vi "Stop.vi"(8 "error in (no error)":errorcluster, 11 "Virt Instr Target in":refnum<class "Virt Instr Target.lvclass">) -> (0 "error out":errorcluster, 3 "Virt Instr Target out":refnum<class "Virt Instr Target.lvclass">)   [LabVIEW 2023, in "HAL GOOP4.lvlib" / "Virt Instr Target.lvclass"]
uses:
  Virt Instr Target.lvclass
  Virt Instr Host/Virt Instr Host.lvclass
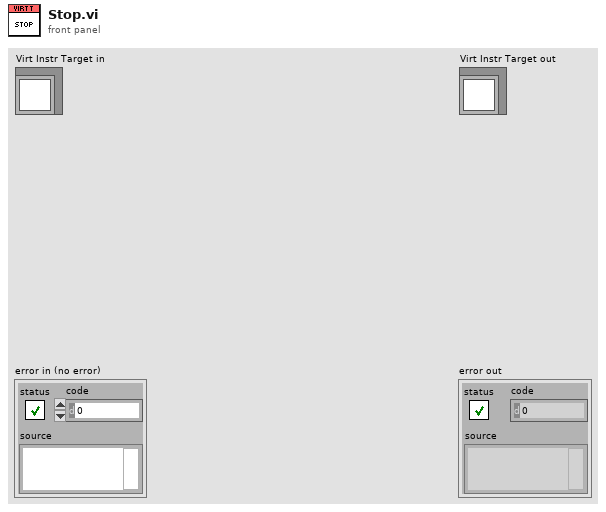
[diagram p1: front panel]
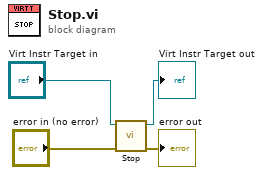
[diagram p0: block diagram]
diagram:
  n1 = call-parent "Stop.vi"("error in (no error)"="error in (no error)", "Virt Instr Base in"="Virt Instr Target in") -> ("error out"=→"error out":errorcluster, "Virt Instr Base out"=→"Virt Instr Target out":refnum<class "Virt Instr Target.lvclass">)  [unwired: 8 in]
